vi "rapid_trace_counts_to_volts.vi"(9 "Offset":dbl, 10 "Channel A Buffer":i16[][](array[numeric]), 11 "Voltage Range":dbl) -> (3 "Voltage Out":dbl[][](array[numeric]))   [LabVIEW 2016]
panel:
  out "Waveform Graph":i16[][](graph)
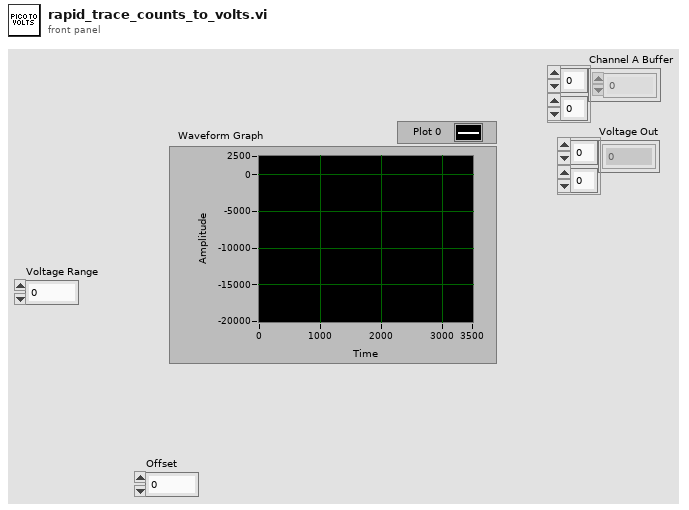
[diagram p1: front panel]
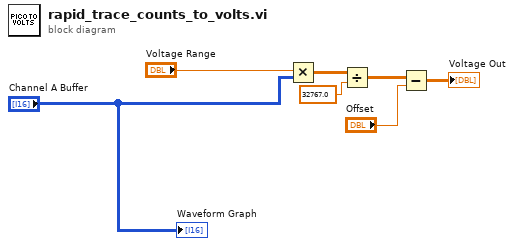
[diagram p0: block diagram]
diagram:
  n1 = Multiply(x="Voltage Range", y="Channel A Buffer") -> (x*y=w6:dbl[][])
  n2 = Divide(x=w6, y=32767.0) -> (x/y=w3:dbl[][])
  n3 = Subtract(x=w3, y="Offset") -> (x-y=→"Voltage Out":dbl[][])
  "Waveform Graph" <- "Channel A Buffer"
